vi "trigger-test2.vi"() -> ()   [LabVIEW 2020]
uses:
  <instrlib>/niDMM/nidmm.llb/niDMM Waveform Function.ctl
  <instrlib>/niDMM/nidmm.llb/niDMM Trigger.ctl
  Realization/PI650 VoltageAmp/TypeDefs/Channel gain.ctl
  Realization/PIPX40 Matrix/PIPX40 Matrix.lvclass
  Realization/PI650 VoltageAmp/PI650 VoltageAmp.lvclass
  Realization/PI650 VoltageAmp/TypeDefs/Channel DC offset.ctl
  Realization/NI Analog Output/NI Analog Output.lvclass
  Realization/NI Analog Output/TypeDefs/Timing Config.ctl
  Realization/NI Analog Output/TypeDefs/Trigger Config.ctl
  Realization/NI DAQmx Base/TypeDefs/Channel Config.ctl
  Realization/NI Analog Input/NI Analog Input.lvclass
  <vilib>/DAQmx/create/channels.llb/DAQmx Create Channel (CO-Pulse Generation-Frequency).vi
  <vilib>/DAQmx/configure/timing.llb/DAQmx Timing (Implicit).vi
  <instrlib>/niDMM/nidmm.llb/niDMM Fetch Waveform (waveform data).vi
  <vilib>/DAQmx/configure/timing.llb/DAQmx Timing (Sample Clock).vi
  <vilib>/DAQmx/configure/trigger.llb/DAQmx Start Trigger (Digital Edge).vi
  <vilib>/measure/NI_MABase.lvlib
  Realization/NI DAQmx Base/NI DAQmx Base.lvclass
  <vilib>/DAQmx/create/channels.llb/DAQmx Create Channel (AO-Voltage-Basic).vi
  <vilib>/DAQmx/write.llb/DAQmx Write (Analog 1D DBL 1Chan NSamp).vi
  <vilib>/DAQmx/read.llb/DAQmx Read (Analog 1D Wfm NChan NSamp).vi
  <vilib>/DAQmx/create/channels.llb/DAQmx Create Channel (AI-Voltage-Basic).vi
panel:
  in  "Channel gain":T1={"Channel (CH1)"=3, "Gain (x1)"=2} {"Channel (CH1)" items=["CH1"=1, "CH2"=2, "CH3"=3, "CH4"=4, "CH5"=5]; "Gain (x1)" items=["x1"=1, "x2"=2, "x5"=3, "x7"=4, "x10"=5, "x14"=6, "x20"=7]}
  out "Amp Info":variant
  out "Mx infos":variant[](array[variant])
  in  "analog input":tag="NI_AnaIn1/ai0:1"
  in  "Trigger Source":T2=enum."TTL 0"
  in  "Function":T3=1003 items=["Waveform_Voltage"=1003, "Waveform_Current"=1004]
  in  "Device Name":refnum<k15>="NI_DMM"
  out "Waveform Graph":dynamicdata(graph)
  in  "counter output":tag="NI_Timing/ctr0"
  out "error out":errorcluster
  in  "source terminal":tag="/NI_Timing/PFI0"
  in  "destination terminal":tag="/NI_AnaIn1/PXI_Trig0"
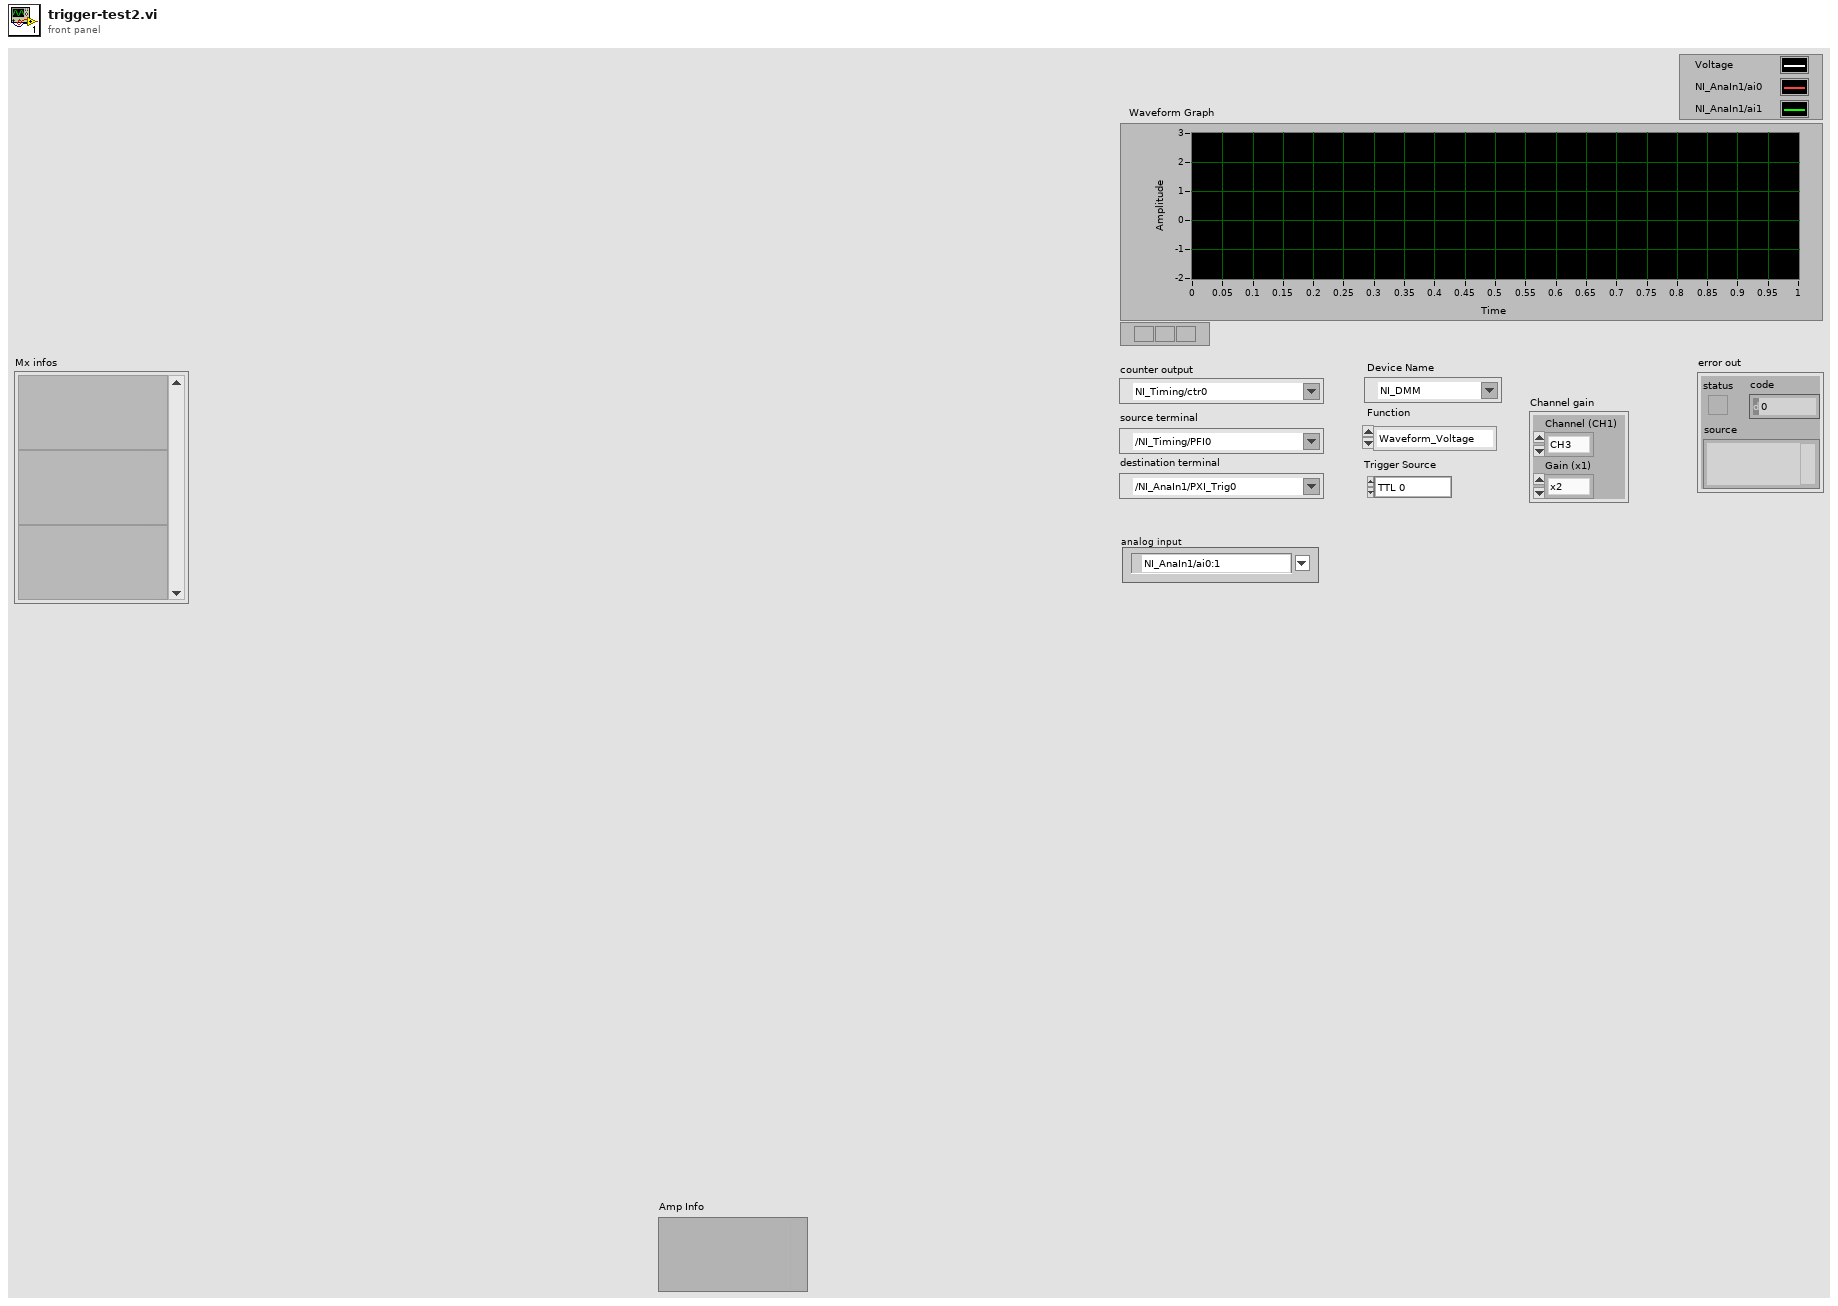
[diagram p1: front panel]
types:
  T1 = typedef "Pickering.lvlib/PI650 VoltageAmp.lvclass/Channel gain.ctl" = cluster{"Channel (CH1)":u32, "Gain (x1)":u32}
  T2 = typedef "niDMM Trigger.ctl" = enum16{"Immediate", "External", "TTL 0", "TTL 1", "TTL 2", "TTL 3", "TTL 4", "TTL 5", "TTL 6", "Software", "TTL 7", "PXI Star", "LBR Trig 1", "Aux Trig 1"}
  T3 = typedef "niDMM Waveform Function.ctl" = i32
  T4 = typedef "Pickering.lvlib/PI650 VoltageAmp.lvclass/Channel DC offset.ctl" = cluster{"Channel (CH1)":u32, "Offset (128)":u32}
  T5 = enum16{"Sine Wave", "Triangle Wave", "Square Wave", "Sawtooth Wave"}
  T6 = map{string, refnum<class "PIPX40 Matrix.lvclass">}
  T7 = cluster{"samples per channel":dbl, "samples per channel":dbl}
  T8 = typedef "NI DAQmx.lvlib/NI DAQmx Base.lvclass/Channel Config.ctl" = cluster{"channels":string, "maximum value":dbl, "minimum value":dbl, "output terminal configuration":i32, "units":i32}
  T9 = typedef "NI DAQmx.lvlib/NI Analog Output.lvclass/Trigger Config.ctl" = cluster{"trigger type":string, "source":string, "slope":i32, "analog level":dbl, "analog hysteresis":dbl}
  T10 = typedef "NI DAQmx.lvlib/NI Analog Output.lvclass/Timing Config.ctl" = cluster{"sample mode":i32, "samples per channel":i32, "rate":dbl, "source":string, "active edge":i32}
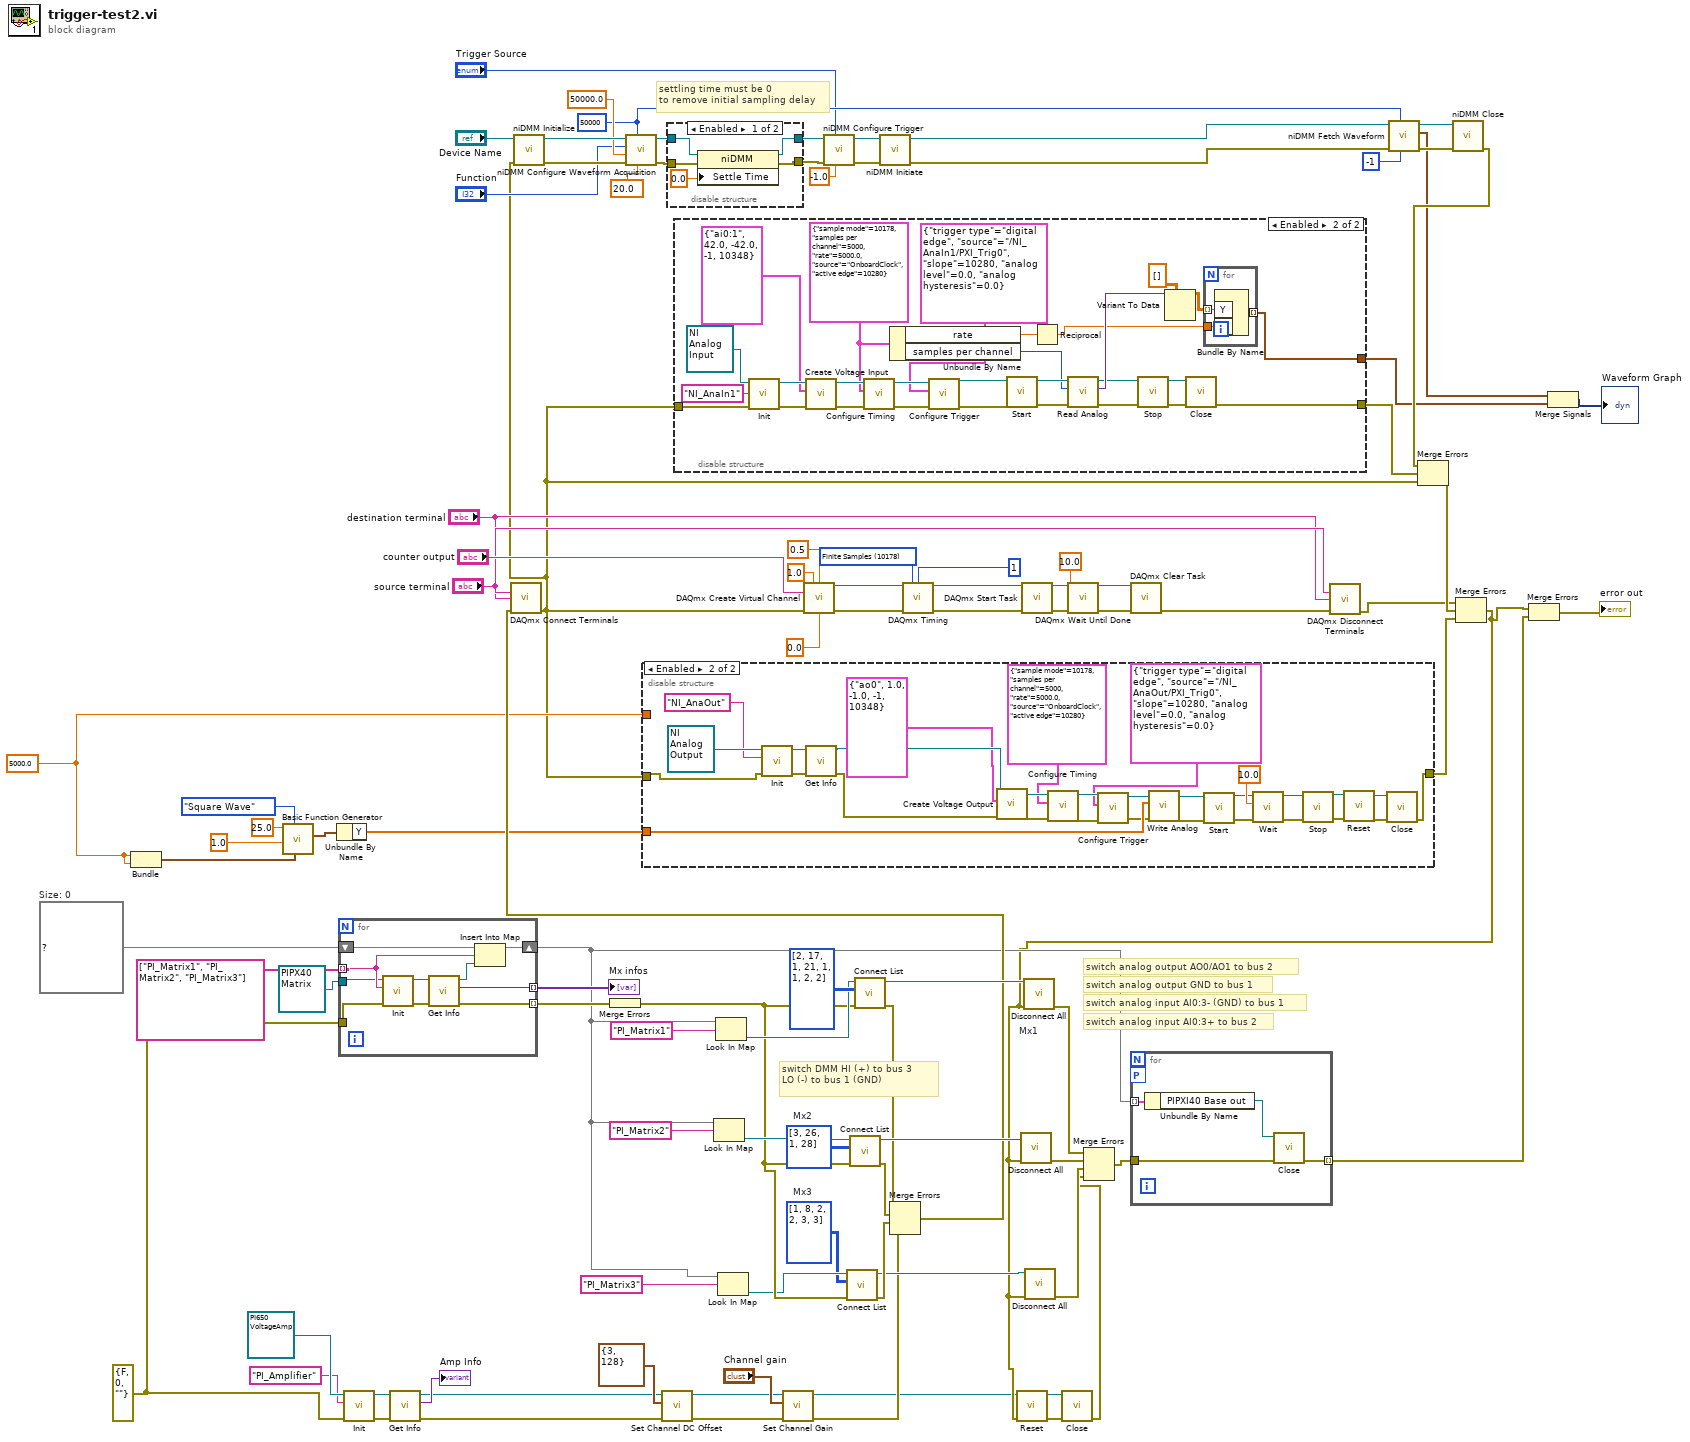
[diagram p0: block diagram]
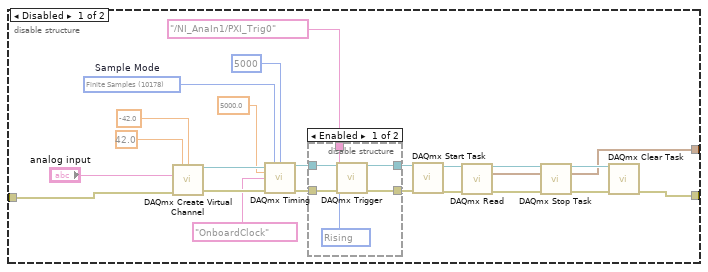
[diagram p3: hidden frame]
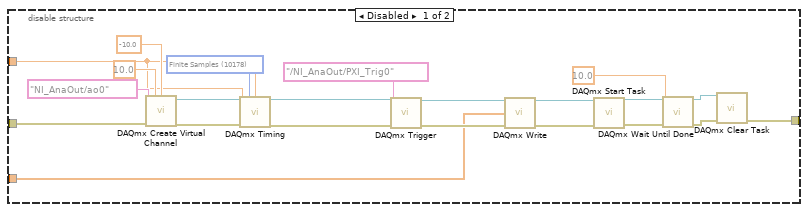
[diagram p5: hidden frame]
diagram:
  w22 = errorcluster {"status"=FALSE, "code"=0, "source"=""} ("error in (no error)")
  w33 = i32[][] [[1, 8], [2, 2], [3, 3]]  # Mx3
  w48 = T6 {}  # Size: 0
  w57 = i32[][] [[3, 26], [1, 28]]  # Mx2
  w59 = i32[][] [[2, 17], [1, 21], [1, 1], [2, 2]]  # Mx1
  w39 = 5000.0 ("samples per channel")
  w71 = 10178 items=["Finite Samples"=10178, "Continuous Samples"=10123, "Hardware Timed Single Point"=12522] ("sample mode")
  w92 = 50000 ("Number of samples")
  # "settling time must be 0\nto remove initial sampling delay"
  # "switch analog input AI0:3+ to bus 2"
  # "switch analog input AI0:3- (GND) to bus 1"
  # "switch analog output GND to bus 1"
  # "switch analog output AO0/AO1 to bus 2"
  # "switch DMM HI (+) to bus 3 \nLO (-) to bus 1 (GND)"
  n1 = Bundle("samples per channel"=w39, "samples per channel"=w39) -> (w38:T7)  [unwired: 1 in]
  n2 = call <vilib>:"Basic Function Generator.vi"("sampling info"=w38, "signal type"=T5."Square Wave", "amplitude"=1.0, "frequency"=25.0) -> ("signal out"=w11:waveform(dbl))  [unwired: 5 in, 2 out]
  n3 = Unbundle By Name(w11) -> ("Y"=w10:dbl[])
  n4 = for {
    tunnel: string[] ["PI_Matrix1", "PI_Matrix2", "PI_Matrix3"] -> [w107] mode=indexing
    tunnel: [w110] -> w62 mode=indexing
    tunnel: [w109] -> w61 mode=indexing
    shift-right: [w108] -> w36
    shift-left: w48 -> [w105]
    tunnel: refnum<class "PIPX40 Matrix.lvclass"> refnum ("PIPXI40 Matrix in") -> [w103]
    tunnel: w22 -> [w102]
    n5 = call-dynamic "Init.vi"("error in (no error)"=w102, "Params"=w107, "PIPXI40 Base in"=w103) -> ("error out"=w111:errorcluster, "PIPXI40 Base out"=w106:refnum<class "PIPX40 Matrix.lvclass">)  [unwired: 7 in]
    n6 = call-dynamic "Get Info.vi"("error in (no error)"=w111, "PIPXI40 Base in"=w106) -> ("error out"=w110:errorcluster, "Info"=w109:variant, "PIPXI40 Base out"=w104:refnum<class "PIPX40 Matrix.lvclass">)  [unwired: 7 in]
    n7 = Insert Into Map(map in=w105, key=w107, value=w104) -> (map out=w108:T6)  [unwired: 2 out]
  }
  "Mx infos" <- w61
  n8 = call-dynamic "Init.vi"("error in (no error)"=w22, "Params"="PI_Amplifier" ("String"), "PI650 VoltageAmp in"=refnum<class "PI650 VoltageAmp.lvclass"> refnum) -> ("error out"=w27:errorcluster, "PI650 VoltageAmp out"=w28:refnum<class "PI650 VoltageAmp.lvclass">)  [unwired: 7 in]
  n9 = call-dynamic "Get Info.vi"("error in (no error)"=w27, "PI650 VoltageAmp in"=w28) -> ("error out"=w21:errorcluster, "Info"=→"Amp Info":variant, "PI650 VoltageAmp out"=w20:refnum<class "PI650 VoltageAmp.lvclass">)  [unwired: 7 in]
  n10 = Merge Errors(w62) -> (w35:errorcluster)
  n11 = call-dynamic "Set Channel DC Offset.vi"("error in (no error)"=w21, "Params"=T4 {"Channel (CH1)"=3, "Offset (128)"=128}, "PI650 VoltageAmp in"=w20) -> ("error out"=w18:errorcluster, "PI650 VoltageAmp out"=w19:refnum<class "PI650 VoltageAmp.lvclass">)  [unwired: 7 in]
  n12 = Look In Map(map=w36, key="PI_Matrix2" ("String")) -> (value=w50:refnum<class "PIPX40 Matrix.lvclass">)  [unwired: 1 in, 1 out]
  n13 = Look In Map(map=w36, key="PI_Matrix1" ("String")) -> (value=w51:refnum<class "PIPX40 Matrix.lvclass">)  [unwired: 1 in, 1 out]
  n14 = Look In Map(map=w36, key="PI_Matrix3" ("String")) -> (value=w34:refnum<class "PIPX40 Matrix.lvclass">)  [unwired: 1 in, 1 out]
  n15 = call-dynamic "Set Channel Gain.vi"("error in (no error)"=w18, "Params"="Channel gain", "PI650 VoltageAmp in"=w19) -> ("error out"=w17:errorcluster, "PI650 VoltageAmp out"=w13:refnum<class "PI650 VoltageAmp.lvclass">)  [unwired: 7 in]
  n16 = call-dynamic "Connect List.vi"("error in (no error)"=w35, "Params"=w33, "PIPXI40 Matrix in"=w34) -> ("error out"=w32:errorcluster, "PIPXI40 Matrix out"=w31:refnum<class "PIPX40 Matrix.lvclass">)  [unwired: 7 in]
  n17 = call-dynamic "Connect List.vi"("error in (no error)"=w35, "Params"=w57, "PIPXI40 Matrix in"=w50) -> ("error out"=w46:errorcluster, "PIPXI40 Matrix out"=w55:refnum<class "PIPX40 Matrix.lvclass">)  [unwired: 7 in]
  n18 = call-dynamic "Connect List.vi"("error in (no error)"=w35, "Params"=w59, "PIPXI40 Matrix in"=w51) -> ("error out"=w47:errorcluster, "PIPXI40 Matrix out"=w56:refnum<class "PIPX40 Matrix.lvclass">)  [unwired: 7 in]
  n19 = Merge Errors(w47, w46, w32, w17) -> (w45:errorcluster)
  n20 = call <vilib>:"DAQmx Connect Terminals.vi"("source terminal"="source terminal", "destination terminal"="destination terminal", "error in"=w45) -> ("error out"=w2:errorcluster)  [unwired: 12 in]
  n21 = call <instrlib>:"niDMM Initialize.vi"("error in (no error)"=w2, "Instrument Descriptor"="Device Name") -> ("error out"=w97:errorcluster, "instrument handle out"=w98:refnum<k15>)  [unwired: 8 in]
  n22 = call <instrlib>:"niDMM Configure Waveform Acquisition.vi"("Range"=20.0, "Waveform Points"=w92, "error in (no error)"=w97, "Rate"=50000.0 ("Sample Rate"), "Function"="Function", "instrument handle"=w98) -> ("error out"=w6:errorcluster, "instrument handle out"=w5:refnum<k15>)  [unwired: 4 in]
  n23 = disable-structure shown="Enabled" {
    disable-tunnel: w2 -> [w132 w158]
    disable-tunnel: [w114 w141] -> w64
    disable-tunnel: w39 -> [w113 _]
    disable-tunnel: w10 -> [w112 w153]
    frame Disabled {
      w127 = 10178 items=["Finite Samples"=10178, "Continuous Samples"=10123, "Hardware Timed Single Point"=12522] ("sample mode")
      n24 = call-poly <vilib>:"DAQmx Create Virtual Channel.vi"("maximum value"=10.0, "minimum value"=-10.0, "physical channels"=tag "NI_AnaOut/ao0", "error in"=w132) -> ("task out"=w128:refnum<k21>, "error out"=w129:errorcluster)  [unwired: 10 in]
      n25 = call-poly <vilib>:"DAQmx Timing.vi"("task/channels in"=w128, "sample mode"=w127, "samples per channel"=w113, "rate"=w113, "error in"=w129) -> ("task out"=w123:refnum<k21>, "error out"=w124:errorcluster)  [unwired: 9 in]
      n26 = call-poly <vilib>:"DAQmx Trigger.vi"("task/channels in"=w123, "source"=tag "/NI_AnaOut/PXI_Trig0", "error in"=w124) -> ("task out"=w121:refnum<k21>, "error out"=w120:errorcluster)  [unwired: 11 in]
      n27 = call-poly <vilib>:"DAQmx Write.vi"("task/channels in"=w121, "data"=w112, "error in"=w120) -> ("task out"=w125:refnum<k21>, "error out"=w126:errorcluster)  [unwired: 10 in, 1 out]
      n28 = call <vilib>:"DAQmx Start Task.vi"("task/channels in"=w125, "error in"=w126) -> ("task out"=w117:refnum<k21>, "error out"=w118:errorcluster)  [unwired: 12 in]
      n29 = call <vilib>:"DAQmx Wait Until Done.vi"("task/channels in"=w117, "timeout (sec)"=10.0, "error in"=w118) -> ("task out"=w116:refnum<k21>, "error out"=w115:errorcluster)  [unwired: 11 in]
      n30 = call <vilib>:"DAQmx Clear Task.vi"("task in"=w116, "error in"=w115) -> ("error out"=w114:errorcluster)  [unwired: 13 in]
    }
    frame Enabled {
      n31 = call-dynamic "Init.vi"("error in (no error)"=w158, "Params"="NI_AnaOut" ("String"), "DAQmx Base in"=refnum<class "NI Analog Output.lvclass"> refnum ("NI DAQmx.lvlib:NI Analog Output.lvclass")) -> ("error out"=w160:errorcluster, "DAQmx Base out"=w161:refnum<class "NI Analog Output.lvclass">)  [unwired: 7 in]
      n32 = call-dynamic "Get Info.vi"("error in (no error)"=w160, "DAQmx Base in"=w161) -> ("error out"=w135:errorcluster, "DAQmx Base out"=w157:refnum<class "NI Analog Output.lvclass">)  [unwired: 7 in, 1 out]
      n33 = call-dynamic "Create Voltage Output.vi"("error in (no error)"=w135, "Params"=T8 {"channels"="ao0", "maximum value"=1.0, "minimum value"=-1.0, "output terminal configuration"=-1, "units"=10348} ("Channel Config"), "NI Analog Output in"=w157) -> ("error out"=w156:errorcluster, "NI Analog Output out"=w155:refnum<class "NI Analog Output.lvclass">)  [unwired: 7 in]
      n34 = call-dynamic "Configure Timing.vi"("error in (no error)"=w156, "Params"=T10 {"sample mode"=10178, "samples per channel"=5000, "rate"=5000.0, "source"="OnboardClock", "active edge"=10280}, "NI DAQmx Base in"=w155) -> ("error out"=w140:errorcluster, "NI DAQmx Base out"=w139:refnum<class "NI Analog Output.lvclass">)  [unwired: 7 in]
      n35 = call-dynamic "Configure Trigger.vi"("error in (no error)"=w140, "Params"=T9 {"trigger type"="digital edge", "source"="/NI_AnaOut/PXI_Trig0", "slope"=10280, "analog level"=0.0, "analog hysteresis"=0.0}, "NI DAQmx Base in"=w139) -> ("error out"=w137:errorcluster, "NI DAQmx Base out"=w138:refnum<class "NI Analog Output.lvclass">)  [unwired: 7 in]
      n36 = call-dynamic "Write Analog.vi"("error in (no error)"=w137, "Params"=w153, "NI Analog Output in"=w138) -> ("error out"=w152:errorcluster, "NI Analog Output out"=w151:refnum<class "NI Analog Output.lvclass">)  [unwired: 7 in]
      n37 = call-dynamic "Start.vi"("error in (no error)"=w152, "NI DAQmx Base in"=w151) -> ("error out"=w145:errorcluster, "NI DAQmx Base out"=w144:refnum<class "NI Analog Output.lvclass">)  [unwired: 8 in]
      n38 = call-dynamic "Wait.vi"("error in (no error)"=w145, "Params"=10.0, "NI DAQmx Base in"=w144) -> ("error out"=w147:errorcluster, "NI DAQmx Base out"=w148:refnum<class "NI Analog Output.lvclass">)  [unwired: 7 in]
      n39 = call-dynamic "Stop.vi"("error in (no error)"=w147, "NI DAQmx Base in"=w148) -> ("error out"=w150:errorcluster, "NI DAQmx Base out"=w149:refnum<class "NI Analog Output.lvclass">)  [unwired: 8 in]
      n40 = call-dynamic "Reset.vi"("error in (no error)"=w150, "DAQmx Base in"=w149) -> ("error out"=w143:errorcluster, "DAQmx Base out"=w142:refnum<class "NI Analog Output.lvclass">)  [unwired: 8 in]
      n41 = call-dynamic "Close.vi"("error in (no error)"=w143, "DAQmx Base in"=w142) -> ("error out"=w141:errorcluster)  [unwired: 8 in, 1 out]
    }
  }
  n42 = disable-structure shown="Enabled" {
    disable-tunnel: w6 -> [w167 w168]
    disable-tunnel: w5 -> [w166 w169]
    disable-tunnel: [w165 w169] -> w4
    disable-tunnel: [w164 w168] -> w3
    frame Enabled {
      n43 = property class="niDMM"(reference=w166, error in=w167, "Settle Time"=0.0 ("Configuration:Advanced:Settle Time")) -> (reference out=w165:refnum<k15>, error out=w164:errorcluster)
    }
    frame Disabled {
    }
  }
  n44 = disable-structure shown="Enabled" {
    disable-tunnel: [w175 w207] -> w65
    disable-tunnel: [w174 w201] -> w1
    disable-tunnel: w2 -> [w170 w221]
    frame Disabled {
      w190 = 10178 items=["Finite Samples"=10178, "Continuous Samples"=10123, "Hardware Timed Single Point"=12522]  # Sample Mode
      n45 = call-poly <vilib>:"DAQmx Create Virtual Channel.vi"("maximum value"=42.0 ("Max Voltage"), "minimum value"=-42.0 ("Min Voltage"), "physical channels"="analog input", "error in"=w170) -> ("task out"=w188:refnum<k21>, "error out"=w189:errorcluster)  [unwired: 10 in]
      n46 = call-poly <vilib>:"DAQmx Timing.vi"("task/channels in"=w188, "sample mode"=w190, "samples per channel"=5000 ("Number of Samples"), "rate"=5000.0 ("Sample Rate"), "source"=tag "OnboardClock" ("Sample Clock Source"), "error in"=w189) -> ("task out"=w192:refnum<k21>, "error out"=w191:errorcluster)  [unwired: 8 in]
      n47 = disable-structure shown="Enabled" {
        disable-tunnel: w192 -> [w198 w200]
        disable-tunnel: w191 -> [w197 w199]
        disable-tunnel: [w196 w200] -> w172
        disable-tunnel: [w195 w199] -> w178
        disable-tunnel: tag "/NI_AnaIn1/PXI_Trig0" ("source") -> [w194 _]
        frame Enabled {
          w193 = 10280 items=["Rising"=10280, "Falling"=10171] ("edge")
          n48 = call-poly <vilib>:"DAQmx Trigger.vi"("task/channels in"=w198, "source"=w194, "edge"=w193, "error in"=w197) -> ("task out"=w196:refnum<k21>, "error out"=w195:errorcluster)  [unwired: 10 in]
        }
        frame Disabled {
        }
      }
      n49 = call <vilib>:"DAQmx Start Task.vi"("task/channels in"=w172, "error in"=w178) -> ("task out"=w171:refnum<k21>, "error out"=w187:errorcluster)  [unwired: 12 in]
      n50 = call-poly <vilib>:"DAQmx Read.vi"("task/channels in"=w171, "error in"=w187) -> ("task out"=w180:refnum<k21>, "data"=w174:waveform(dbl)[], "error out"=w179:errorcluster)  [unwired: 11 in]
      n51 = call <vilib>:"DAQmx Stop Task.vi"("task/channels in"=w180, "error in"=w179) -> ("task out"=w182:refnum<k21>, "error out"=w181:errorcluster)  [unwired: 12 in]
      n52 = call <vilib>:"DAQmx Clear Task.vi"("task in"=w182, "error in"=w181) -> ("error out"=w175:errorcluster)  [unwired: 13 in]
    }
    frame Enabled {
      w205 = T10 {"sample mode"=10178, "samples per channel"=5000, "rate"=5000.0, "source"="OnboardClock", "active edge"=10280}
      n53 = call-dynamic "Init.vi"("error in (no error)"=w221, "Params"="NI_AnaIn1" ("String"), "DAQmx Base in"=refnum<class "NI Analog Input.lvclass"> refnum ("NI Analog Input in")) -> ("error out"=w227:errorcluster, "DAQmx Base out"=w226:refnum<class "NI Analog Input.lvclass">)  [unwired: 7 in]
      n54 = call-dynamic "Create Voltage Input.vi"("error in (no error)"=w227, "Params"=T8 {"channels"="ai0:1", "maximum value"=42.0, "minimum value"=-42.0, "output terminal configuration"=-1, "units"=10348} ("Channel Config"), "NI Analog Input in"=w226) -> ("error out"=w228:errorcluster, "NI Analog Input out"=w225:refnum<class "NI Analog Input.lvclass">)  [unwired: 7 in]
      n55 = call-dynamic "Configure Timing.vi"("error in (no error)"=w228, "Params"=w205, "NI DAQmx Base in"=w225) -> ("error out"=w223:errorcluster, "NI DAQmx Base out"=w224:refnum<class "NI Analog Input.lvclass">)  [unwired: 7 in]
      n56 = Unbundle By Name(w205) -> ("rate"=w203:dbl, "samples per channel"=w204:i32)
      n57 = call-dynamic "Configure Trigger.vi"("error in (no error)"=w223, "Params"=T9 {"trigger type"="digital edge", "source"="/NI_AnaIn1/PXI_Trig0", "slope"=10280, "analog level"=0.0, "analog hysteresis"=0.0}, "NI DAQmx Base in"=w224) -> ("error out"=w216:errorcluster, "NI DAQmx Base out"=w215:refnum<class "NI Analog Input.lvclass">)  [unwired: 7 in]
      n58 = call-dynamic "Start.vi"("error in (no error)"=w216, "NI DAQmx Base in"=w215) -> ("error out"=w217:errorcluster, "NI DAQmx Base out"=w214:refnum<class "NI Analog Input.lvclass">)  [unwired: 8 in]
      n59 = Reciprocal(x=w203) -> (1/x=w202:dbl)
      n60 = call-dynamic "Read Analog.vi"("error in (no error)"=w217, "Params"=w204, "NI Analog Input in"=w214) -> ("error out"=w209:errorcluster, "Data"=w212:variant, "NI Analog Input out"=w210:refnum<class "NI Analog Input.lvclass">)  [unwired: 6 in]
      n61 = call-dynamic "Stop.vi"("error in (no error)"=w209, "NI DAQmx Base in"=w210) -> ("error out"=w208:errorcluster, "NI DAQmx Base out"=w211:refnum<class "NI Analog Input.lvclass">)  [unwired: 8 in]
      n62 = Variant To Data(type=dbl[][] [], Variant=w212) -> (data=w206:dbl[][])  [unwired: 1 in, 1 out]
      n63 = call-dynamic "Close.vi"("error in (no error)"=w208, "DAQmx Base in"=w211) -> ("error out"=w207:errorcluster)  [unwired: 8 in, 1 out]
      n64 = for {
        tunnel: w206 -> [w231] mode=indexing
        tunnel: [w230] -> w201 mode=indexing
        tunnel: w202 -> [w229]
        n65 = Bundle By Name("Y"=w231, "dt"=w229) -> (w230:waveform(dbl))  [unwired: 1 in]
      }
    }
  }
  n66 = call-poly <vilib>:"DAQmx Create Virtual Channel.vi"("frequency"=1.0, "duty cycle"=0.5, "counter"="counter output", "error in"=w2, "initial delay"=0.0) -> ("task out"=w69:refnum<k21>, "error out"=w70:errorcluster)  [unwired: 9 in]
  n67 = call <instrlib>:"niDMM Configure Trigger.vi"("Trigger Delay (sec)"=-1.0, "Trigger Source"="Trigger Source", "error in (no error)"=w3, "instrument handle"=w4) -> ("error out"=w89:errorcluster, "instrument handle out"=w90:refnum<k15>)  [unwired: 6 in]
  n68 = call <instrlib>:"niDMM Initiate.vi"("error in (no error)"=w89, "instrument handle"=w90) -> ("error out"=w87:errorcluster, "instrument handle out"=w7:refnum<k15>)  [unwired: 8 in]
  n69 = call-poly <vilib>:"DAQmx Timing.vi"("task/channels in"=w69, "sample mode"=w71, "samples per channel"=1, "error in"=w70) -> ("task out"=w79:refnum<k21>, "error out"=w80:errorcluster)  [unwired: 10 in]
  n70 = call <vilib>:"DAQmx Start Task.vi"("task/channels in"=w79, "error in"=w80) -> ("task out"=w77:refnum<k21>, "error out"=w78:errorcluster)  [unwired: 12 in]
  n71 = call <vilib>:"DAQmx Wait Until Done.vi"("task/channels in"=w77, "timeout (sec)"=10.0, "error in"=w78) -> ("task out"=w8:refnum<k21>, "error out"=w81:errorcluster)  [unwired: 11 in]
  n72 = call <vilib>:"DAQmx Clear Task.vi"("task in"=w8, "error in"=w81) -> ("error out"=w82:errorcluster)  [unwired: 13 in]
  n73 = call <vilib>:"DAQmx Disconnect Terminals.vi"("source terminal"="source terminal", "destination terminal"="destination terminal", "error in"=w82) -> ("error out"=w83:errorcluster)  [unwired: 12 in]
  n74 = call-poly <instrlib>:"niDMM Fetch Waveform.vi"("Maximum Time (msec)"=-1, "Number To Fetch"=w92, "error in (no error)"=w87, "instrument handle"=w7) -> ("error out"=w88:errorcluster, "Waveform Data"=w84:waveform(dbl), "instrument handle out"=w91:refnum<k15>)  [unwired: 4 in, 1 out]
  n75 = call <instrlib>:"niDMM Close.vi"("error in (no error)"=w88, "instrument handle"=w91) -> ("error out"=w85:errorcluster)  [unwired: 9 in]
  n76 = Merge Errors(w85, w65, w2) -> (w100:errorcluster)
  n77 = Merge Errors(w83, w100, w64) -> (w14:errorcluster)
  n78 = call-dynamic "Reset.vi"("error in (no error)"=w14, "PI650 VoltageAmp in"=w13) -> ("error out"=w15:errorcluster, "PI650 VoltageAmp out"=w16:refnum<class "PI650 VoltageAmp.lvclass">)  [unwired: 8 in]
  n79 = call-dynamic "Disconnect All.vi"("error in (no error)"=w14, "PIPXI40 Matrix in"=w55) -> ("error out"=w54:errorcluster)  [unwired: 8 in, 1 out]
  n80 = call-dynamic "Disconnect All.vi"("error in (no error)"=w14, "PIPXI40 Matrix in"=w56) -> ("error out"=w53:errorcluster)  [unwired: 8 in, 1 out]
  n81 = call-dynamic "Disconnect All.vi"("error in (no error)"=w14, "PIPXI40 Matrix in"=w31) -> ("error out"=w30:errorcluster)  [unwired: 8 in, 1 out]
  n82 = call-dynamic "Close.vi"("error in (no error)"=w15, "PI650 VoltageAmp in"=w16) -> ("error out"=w12:errorcluster)  [unwired: 8 in, 1 out]
  n83 = Merge Errors(w53, w54, w30, w12) -> (w52:errorcluster)
  n84 = for {
    tunnel: w52 -> [w234]
    tunnel: [w235] -> w44 mode=indexing
    workers-P: _ -> [_]
    tunnel: w36 -> [w233] mode=indexing
    n85 = Unbundle By Name(w233) -> ("PIPXI40 Base out"=w232:refnum<class "PIPX40 Matrix.lvclass">)
    n86 = call-dynamic "Close.vi"("error in (no error)"=w234, "PIPXI40 Base in"=w232) -> ("error out"=w235:errorcluster)  [unwired: 8 in, 1 out]
  }
  n87 = Merge Errors(w14, w44) -> (→"error out":errorcluster)
  n88 = Merge Signals(w84, w1) -> (→"Waveform Graph":dynamicdata)
